vi "루프 안에 두개.vi"() -> ()   [LabVIEW 2020]
uses:
  <vilib>/userdefined/High Color/IMAQdx.ctl
  <vilib>/vision/driver/IMAQdx.llb/IMAQdx Acquisition Mode.ctl
  <vilib>/vision/driver/IMAQdx.llb/IMAQdx Buffer Number Mode.ctl
  <vilib>/vision/driver/NI_Vision_Acquisition_Software.lvlib
  <resource>/objmgr/imaqdx.rc
panel:
  out "Buffer Number Out 2":u32
  out "Images Missed 2":u32
  out "Images Behind 2":i32
  out "Processed Frames per Second 2":dbl
  out "Acquired Frames per Second 2":dbl
  out "Image 2":T1(plugin-control) caption="Image"
  in  "IMAQdx Session 2":T2
  in  "Stop Stream":bool
  in  "Simulated Processing Delay (ms)":i32
  out "Buffer Number Out":u32
  out "Images Missed":u32
  out "Images Behind":i32
  out "Processed Frames per Second":dbl
  out "Acquired Frames per Second":dbl
  out "Image":T1(plugin-control)
  in  "Number of Images (err Iteration)":i32
  in  "OverwriteMode":u16(ring) items=["Get Oldest"=0, "Fail"=2, "Get Newest"=3]
  in  "IMAQdx Session":T2
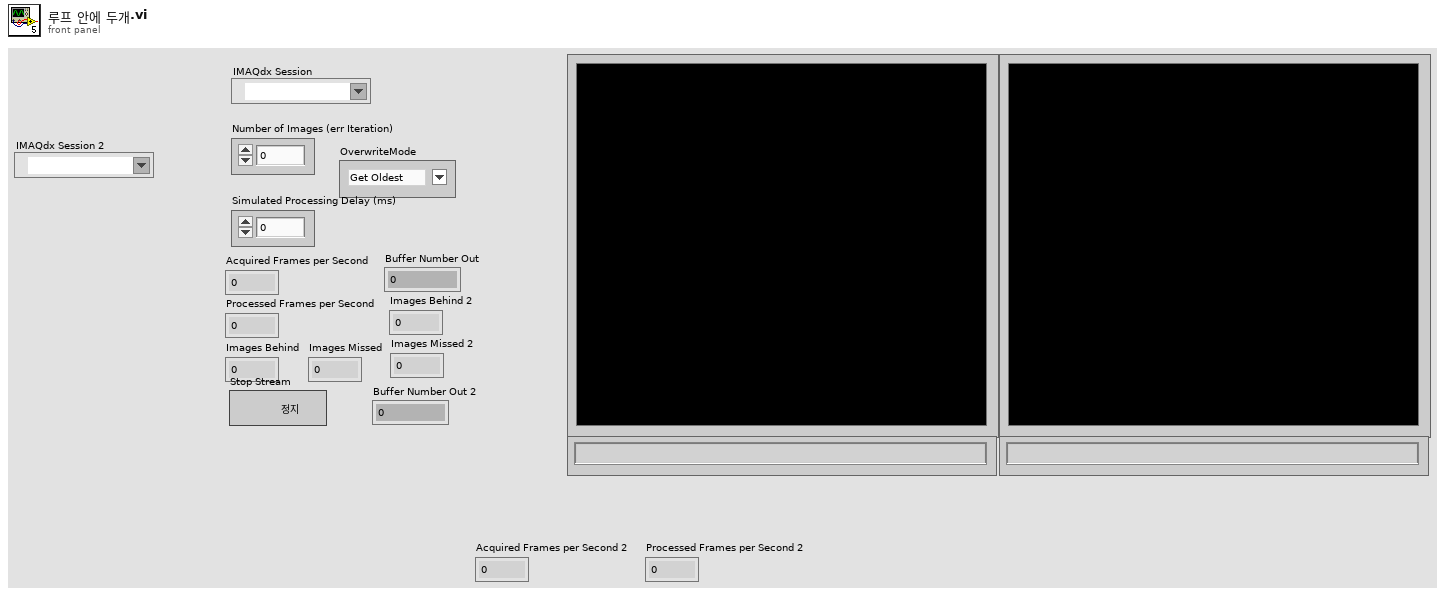
[diagram p1: front panel]
types:
  T1 = typedef "IMAQ Image.ctl" = refnum<image>
  T2 = typedef "IMAQdx.ctl" = refnum<k21>
  T3 = typedef "NI_Vision_Acquisition_Software.lvlib/IMAQdx Acquisition Mode.ctl" = enum32{"One Shot", "Continuous"}
  T4 = typedef "NI_Vision_Acquisition_Software.lvlib/IMAQdx Buffer Number Mode.ctl" = enum32{"Next", "Last", "Buffer Number", "Every", "Last New"}
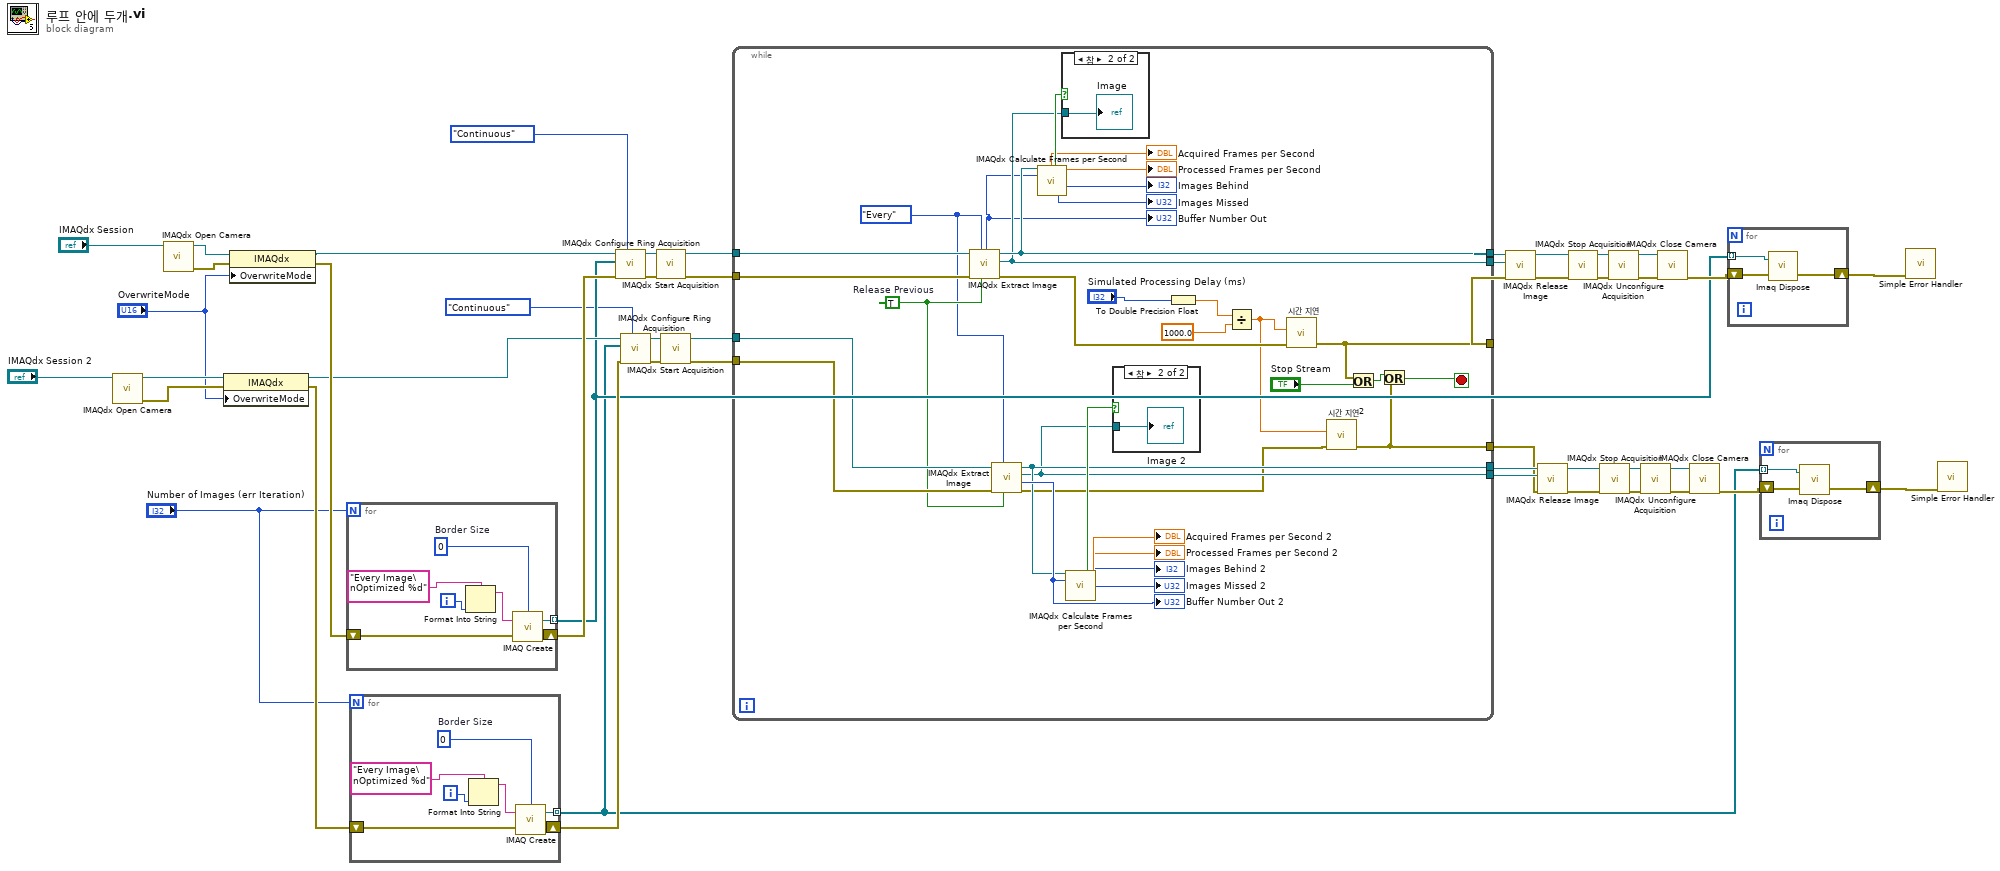
[diagram p0: block diagram]
diagram:
  n1 = call <vilib>:"IMAQdx Open Camera.vi"("Session In"="IMAQdx Session 2") -> ("error out"=w25:errorcluster, "Session Out"=w26:T2)  [unwired: 9 in]
  n2 = call <vilib>:"IMAQdx Open Camera.vi"("Session In"="IMAQdx Session") -> ("error out"=w46:errorcluster, "Session Out"=w47:T2)  [unwired: 9 in]
  n3 = property class="IMAQdx"(reference=w26, error in=w25, "OverwriteMode"="OverwriteMode") -> (reference out=w18:T2, error out=w23:errorcluster)
  n4 = property class="IMAQdx"(reference=w47, error in=w46, "OverwriteMode"="OverwriteMode") -> (reference out=w44:T2, error out=w45:errorcluster)
  n5 = for {
    N: "Number of Images (err Iteration)" -> [_]
    tunnel: [w51] -> w14 mode=indexing
    shift-right: [w49] -> w43
    shift-left: w45 -> [w50]
    i -> [w54]
    w52 = 0  # Border Size
    n6 = Format Into String(format string="Every Image\nOptimized %d", w54) -> (resulting string=w53:string)  [unwired: 2 in, 1 out]
    n7 = call "IMAQ Create"("Border Size"=w52, "Image Name"=w53, "error in (no error)"=w50) -> ("New Image"=w51:T1, "error out"=w49:errorcluster)  [unwired: 2 in]
  }
  n8 = for {
    N: "Number of Images (err Iteration)" -> [_]
    tunnel: [w58] -> w5 mode=indexing
    shift-right: [w56] -> w21
    shift-left: w23 -> [w57]
    i -> [w61]
    w59 = 0  # Border Size
    n9 = Format Into String(format string="Every Image\nOptimized %d", w61) -> (resulting string=w60:string)  [unwired: 2 in, 1 out]
    n10 = call "IMAQ Create"("Border Size"=w59, "Image Name"=w60, "error in (no error)"=w57) -> ("New Image"=w58:T1, "error out"=w56:errorcluster)  [unwired: 2 in]
  }
  n11 = call <vilib>:"IMAQdx Configure Ring Acquisition.vi"("Mode"=IMAQdx_Acquisition_Mode."Continuous", "error in"=w43, "Images"=w14, "Session In"=w44) -> ("error out"=w41:errorcluster, "Session Out"=w42:T2)  [unwired: 5 in, 1 out]
  n12 = call <vilib>:"IMAQdx Configure Ring Acquisition.vi"("Mode"=IMAQdx_Acquisition_Mode."Continuous", "error in"=w21, "Images"=w5, "Session In"=w18) -> ("error out"=w19:errorcluster, "Session Out"=w20:T2)  [unwired: 5 in, 1 out]
  n13 = call <vilib>:"IMAQdx Start Acquisition.vi"("error in"=w41, "Session In"=w42) -> ("error out"=w40:errorcluster, "Session Out"=w39:T2)  [unwired: 8 in]
  n14 = call <vilib>:"IMAQdx Start Acquisition.vi"("error in"=w19, "Session In"=w20) -> ("error out"=w16:errorcluster, "Session Out"=w17:T2)  [unwired: 8 in]
  n15 = while {
    tunnel: w40 -> [w87]
    tunnel: w39 -> [w95]
    tunnel: [w84] -> w36
    tunnel: [w83] -> w38
    tunnel: [w82] -> w37
    tunnel: w17 -> [w81]
    tunnel: w16 -> [w80]
    tunnel: [w70] -> w4
    tunnel: [w69] -> w3
    tunnel: [w63] -> w2
    stop <- w64 stop-if-true
    w79 = TRUE  # Release Previous
    w78 = IMAQdx_Buffer_Number_Mode."Every" ("Buffer Number Mode (Next)")
    n16 = call <vilib>:"IMAQdx Extract Image.vi"("Release Previous (true)"=w79, "Buffer Number Mode (Next)"=w78, "error in"=w87, "Session In"=w95) -> ("error out"=w93:errorcluster, "Buffer Number Out"=w73:u32, "Image Out"=w82:T1, "Session Out"=w83:T2)  [unwired: 4 in]
    "Buffer Number Out" <- w73
    n17 = call <vilib>:"IMAQdx Extract Image.vi"("Release Previous (true)"=w79, "Buffer Number Mode (Next)"=w78, "error in"=w80, "Session In"=w81) -> ("error out"=w66:errorcluster, "Buffer Number Out"=w71:u32, "Image Out"=w69:T1, "Session Out"=w70:T2)  [unwired: 4 in]
    "Buffer Number Out 2" <- w71
    n18 = call <vilib>:"IMAQdx Calculate Frames per Second.vi"("Session In"=w83, "Buffer Number"=w73) -> ("Update Display"=w94:bool, "Acquired Frames per Second"=→"Acquired Frames per Second":dbl, "Processed Frames per Second"=→"Processed Frames per Second":dbl, "Images Behind"=→"Images Behind":i32, "Images Missed"=→"Images Missed":u32)  [unwired: 7 in, 2 out]
    n19 = case shown="참" w94 {
      tunnel: w82 -> [_ w97]
      frame False {
      }
      frame True {
        "Image" <- w97
      }
    }
    n20 = call <vilib>:"IMAQdx Calculate Frames per Second.vi"("Session In"=w70, "Buffer Number"=w71) -> ("Update Display"=w77:bool, "Acquired Frames per Second"=→"Acquired Frames per Second 2":dbl, "Processed Frames per Second"=→"Processed Frames per Second 2":dbl, "Images Behind"=→"Images Behind 2":i32, "Images Missed"=→"Images Missed 2":u32)  [unwired: 7 in, 2 out]
    n21 = case shown="참" w77 {
      tunnel: w69 -> [_ w96]
      frame False {
      }
      frame True {
        "Image 2" <- w96
      }
    }
    n22 = To Double Precision Float(number="Simulated Processing Delay (ms)") -> (double precision float=w86:dbl)
    n23 = Divide(x=w86, y=1000.0) -> (x/y=w67:dbl)
    n24 = call "시간 지연"("error in (no error)"=w93, "Delay Time (s)"=w67) -> ("error out"=w84:errorcluster)  [unwired: 9 in]
    n25 = call "시간 지연2"("error in (no error)"=w66, "Delay Time (s)"=w67) -> ("error out"=w63:errorcluster)  [unwired: 9 in]
    n26 = Or(x=w84, y="Stop Stream") -> (x .or. y?=w65:bool)
    n27 = Or(x=w65, y=w63) -> (x .or. y?=w64:bool)
  }
  n28 = call <vilib>:"IMAQdx Release Image.vi"("error in"=w36, "Image"=w37, "Session In"=w38) -> ("error out"=w34:errorcluster, "Session Out"=w35:T2)  [unwired: 7 in]
  n29 = call <vilib>:"IMAQdx Release Image.vi"("error in"=w2, "Image"=w3, "Session In"=w4) -> ("error out"=w12:errorcluster, "Session Out"=w13:T2)  [unwired: 7 in]
  n30 = call <vilib>:"IMAQdx Stop Acquisition.vi"("error in"=w34, "Session In"=w35) -> ("error out"=w33:errorcluster, "Session Out"=w32:T2)  [unwired: 8 in]
  n31 = call <vilib>:"IMAQdx Stop Acquisition.vi"("error in"=w12, "Session In"=w13) -> ("error out"=w11:errorcluster, "Session Out"=w10:T2)  [unwired: 8 in]
  n32 = call <vilib>:"IMAQdx Unconfigure Acquisition.vi"("error in"=w33, "Session In"=w32) -> ("error out"=w30:errorcluster, "Session Out"=w31:T2)  [unwired: 8 in]
  n33 = call <vilib>:"IMAQdx Unconfigure Acquisition.vi"("error in"=w11, "Session In"=w10) -> ("error out"=w8:errorcluster, "Session Out"=w9:T2)  [unwired: 8 in]
  n34 = call <vilib>:"IMAQdx Close Camera.vi"("error in"=w30, "Session In"=w31) -> ("error out"=w28:errorcluster)  [unwired: 9 in]
  n35 = call <vilib>:"IMAQdx Close Camera.vi"("error in"=w8, "Session In"=w9) -> ("error out"=w6:errorcluster)  [unwired: 9 in]
  n36 = for {
    tunnel: w14 -> [w100] mode=indexing
    shift-right: [w99] -> w29
    shift-left: w28 -> [w98]
    n37 = call "Imaq Dispose"("Image"=w100, "error in (no error)"=w98) -> ("error out"=w99:errorcluster)  [unwired: 4 in]
  }
  n38 = for {
    tunnel: w5 -> [w103] mode=indexing
    shift-right: [w102] -> w7
    shift-left: w6 -> [w101]
    n39 = call "Imaq Dispose"("Image"=w103, "error in (no error)"=w101) -> ("error out"=w102:errorcluster)  [unwired: 4 in]
  }
  n40 = call <vilib>:"Simple Error Handler.vi"("error in (no error)"=w29) -> ()  [unwired: 4 in, 5 out]
  n41 = call <vilib>:"Simple Error Handler.vi"("error in (no error)"=w7) -> ()  [unwired: 4 in, 5 out]
